vi "Synchronization.vi"() -> ()   [LabVIEW 2021]
panel:
  out "Waveform Chart 2":dbl(graph)
  out "Waveform Chart":dbl(graph)
  in  "stop":bool
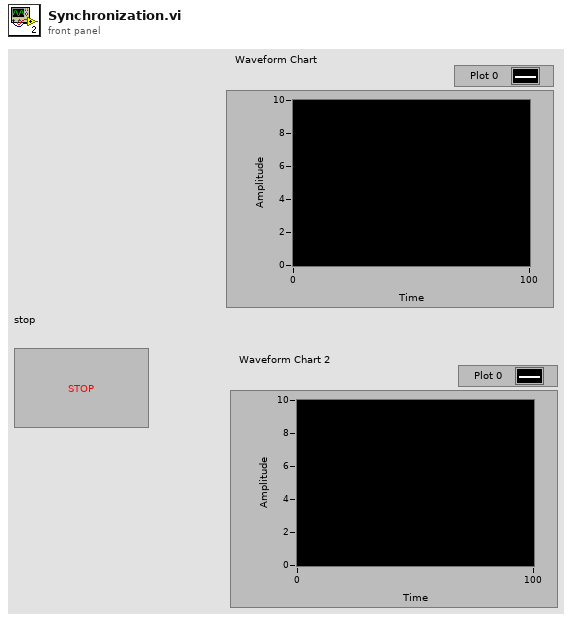
[diagram p1: front panel]
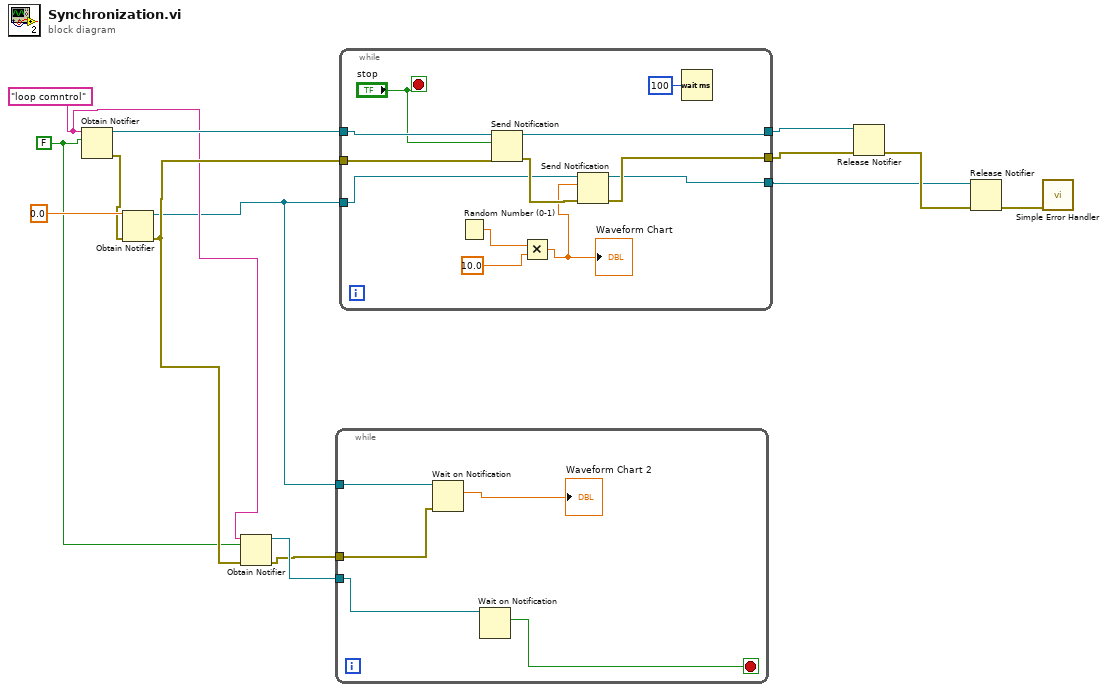
[diagram p0: block diagram]
diagram:
  w3 = "loop comntrol" ("name (unnamed)")
  w1 = FALSE
  n1 = Obtain Notifier(name (unnamed)=w3, notification data type=w1) -> (notifier out=w14:refnum<notifier>, error out=w6:errorcluster)  [unwired: 2 in, 1 out]
  n2 = Obtain Notifier(notification data type=0.0, error in (no error)=w6) -> (notifier out=w2:refnum<notifier>, error out=w5:errorcluster)  [unwired: 2 in, 1 out]
  n3 = Obtain Notifier(name (unnamed)=w3, notification data type=w1, error in (no error)=w5) -> (notifier out=w8:refnum<notifier>, error out=w4:errorcluster)  [unwired: 1 in, 1 out]
  n4 = while {
    tunnel: w8 -> [w17]
    tunnel: w4 -> [w19]
    tunnel: w2 -> [w16]
    stop <- w18 stop-if-true
    n5 = Wait on Notification(notifier=w16, error in (no error)=w19) -> (notification=→"Waveform Chart 2":dbl)  [unwired: 2 in, 3 out]
    n6 = Wait on Notification(notifier=w17) -> (notification=w18:bool)  [unwired: 3 in, 3 out]
  }
  n7 = while {
    tunnel: w14 -> [w31]
    tunnel: w5 -> [w29]
    tunnel: [w27] -> w12
    tunnel: [w26] -> w13
    tunnel: w2 -> [w25]
    tunnel: [w24] -> w10
    stop <- "stop" stop-if-true
    n8 = Random Number (0-1)() -> (number: 0 to 1=w23:dbl)
    n9 = Send Notification(notification="stop", notifier=w31, error in (no error)=w29) -> (notifier out=w26:refnum<notifier>, error out=w28:errorcluster)
    n10 = Multiply(x=w23, y=10.0) -> (x*y=w21:dbl)
    "Waveform Chart" <- w21
    n11 = Send Notification(notification=w21, notifier=w25, error in (no error)=w28) -> (notifier out=w24:refnum<notifier>, error out=w27:errorcluster)
    n12 = Wait (ms)(milliseconds to wait=u32 100) -> ()  [unwired: 1 out]
  }
  n13 = Release Notifier(notifier=w13, error in (no error)=w12) -> (error out=w11:errorcluster)  [unwired: 1 in, 2 out]
  n14 = Release Notifier(notifier=w10, error in (no error)=w11) -> (error out=w9:errorcluster)  [unwired: 1 in, 2 out]
  n15 = call <vilib>:"Simple Error Handler.vi"("error in (no error)"=w9) -> ()  [unwired: 4 in, 5 out]
